vi "Begins_With.vi"(2 "Beginning":string, 3 "String":string) -> (0 "Beginning To Large?":bool, 1 "Begins With?":bool)   [LabVIEW 2016]
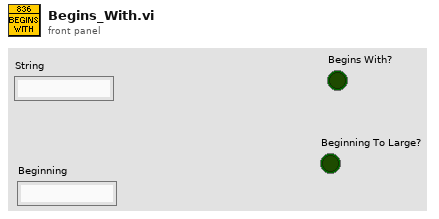
[diagram p1: front panel]
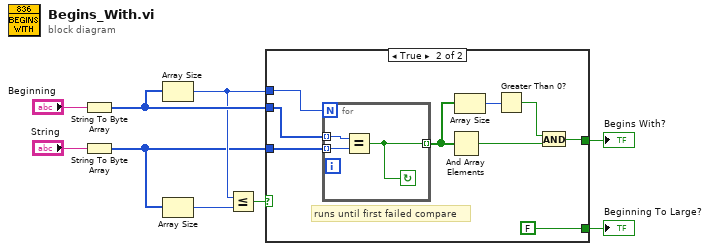
[diagram p0: block diagram]
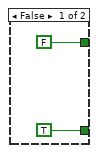
[diagram p2: hidden frame]
diagram:
  n1 = String To Byte Array(string="Beginning") -> (unsigned byte array=w7:u8[])
  n2 = String To Byte Array(string="String") -> (unsigned byte array=w5:u8[])
  n3 = Array Size(array=w7) -> (size(s)=w6:i32)
  n4 = Array Size(array=w5) -> (size(s)=w4:i32)
  n5 = Less Or Equal?(x=w6, y=w4) -> (x <= y?=w3:bool)
  n6 = case shown="True" w3 {
    tunnel: w6 -> [_ w20]
    tunnel: w7 -> [_ w19]
    tunnel: w5 -> [_ w18]
    tunnel: [FALSE w15] -> w2
    tunnel: [TRUE FALSE] -> w1
    frame False {
    }
    frame True {
      # "runs until first failed compare"
      n7 = for {
        N: w20 -> [_]
        tunnel: w19 -> [w23] mode=indexing
        tunnel: w18 -> [w22] mode=indexing
        tunnel: [w21] -> w16 mode=indexing
        stop <- w21 continue-if-true
        n8 = Equal?(x=w23, y=w22) -> (x = y?=w21:bool)
      }
      n9 = And Array Elements(Boolean array=w16) -> (logical AND=w14:bool)
      n10 = Array Size(array=w16) -> (size(s)=w13:i32)
      n11 = Greater Than 0?(x=w13) -> (x > 0?=w12:bool)
      n12 = And(x=w12, y=w14) -> (x .and. y?=w15:bool)
    }
  }
  "Begins With?" <- w2
  "Beginning To Large?" <- w1
